vi "LEDstateintensity.vi"(8 "error in (no error)":errorcluster, 9 "intensity":u8, 10 "port":i16, 11 "Id":i16) -> (0 "error out":errorcluster, 2 "port out":i16, 3 "Id out":i16)   [LabVIEW 2015]
uses:
  PacDriveSDK/C#/bin/Debug/PacDrive32.dll
panel:
  out "return type":u8
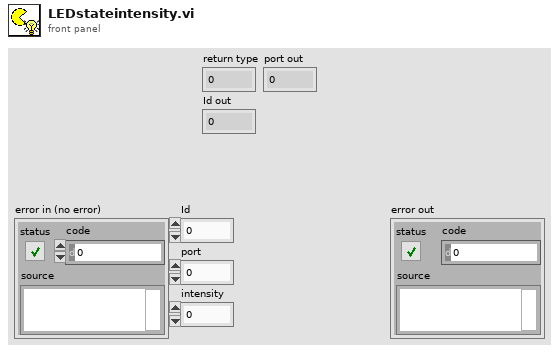
[diagram p1: front panel]
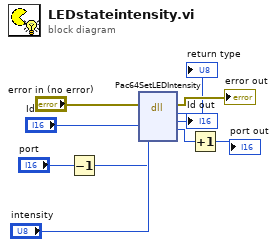
[diagram p0: block diagram]
diagram:
  n1 = Decrement(x="port") -> (x-1=w4:i16)
  n2 = dll-call lib="C:/Users/Team4153/Documents/GitHub/2016_competition/2016 Dashboard Project/TestLights Folder/PacDriveSDK/C#/bin/Debug/PacDrive32.dll" fn="Pac64SetLEDIntensity"(error in="error in (no error)", "Id"="Id", "port"=w4, "intensity"="intensity") -> (error out=→"error out":errorcluster, "return type"=→"return type":u8, "Id"=→"Id out":i16, "port"=w2:i16)  [unwired: 3 in, 1 out]
  n3 = Increment(x=w2) -> (x+1=→"port out":i16)
